vi "Read Waveform Measurement One Channel.vi"(4 "Measurement Type (0: Statistic Average)":u16(ring) items=["Statistic Average", "Current Statistic Value", "Statistic Maximum", "Statistic Minimum", "Statistic Standard Deviation", "Counter"], 6 "Measurement Function (0: Falling Edge)":u16(ring) items=["Waveform Peak-Peak Value", "Waveform Amplitude Value", "Waveform Maximum", "Waveform Minimum", "Waveform Top Value", "Waveform Amplitude Base Value", "Rover Shoot", "Fover Shoot", "RPre Shoot", "FPre Shoot", "Waveform Amplitude Average(Display)", "Waveform Amplitude Average(Cycle)", "Waveform RMS(DC Display)", "Waveform RMS(DC Cycle)", "Waveform RMS(AC Display)", "Waveform RMS(AC Cycle)", "Waveform Adjust Mean", "Period", "Frequency", "Raising Time", "Fall Time", "Positive Pulse", "Negative Pulse", "Positive Duty", "Negative Duty", "Burst Width", "PulSetrain", "XMax", "XMin", "Setup Time", "Hold Time", "ShRatio", "Baud", "Raising Count", "Falling Count", "Positive Count", "Negtive Count", "Triger Count", "Area (Display)", "Area(Cycle)", "Positvie Area(Display)", "Positive Area(Cycle)", "Negtive Area(Display)", "Negtive Area(Cycle)"], 7 "Channel (1: Channel 1)":u16(ring)=1 items=["Channel 1"=1, "Channel 2"=2, "Channel 3"=3, "Channel 4"=4], 8 "error in (no error)":errorcluster, 10 "Timeout (1000 ms)":dbl=1000.0, 11 "VISA resource name":refnum<visa-resource-name>) -> (0 "error out":errorcluster, 2 "Measurement":dbl, 3 "VISA resource name out":refnum<visa-resource-name>)   [LabVIEW 2015, in "ZhiYuan ZDS Series for TCP.lvlib"]
doc: "Returns the waveform the oscilloscope acquired for the specified channel. The waveform is from an acquisition that you initiate prior to calling this VI.\n\nYou use the Initiate VI to start an acquisition on the channels that you enable with the Configure Channel VI. The oscilloscope acquires waveforms for the enabled channels concurrently. You must call this VI separately for each enabled channel to obtain the waveforms.\n\nYou can call the Read Waveform VI instead of using low-level VIs.\n\n<B>Note:</B> Use this VI only with other low-level VIs. The high-level VIs automatically incorporate this functionality. This VI does not check the instrument status."
uses:
  ZhiYuan ZDS Series for TCP.lvlib
panel:
  out "字符串":string
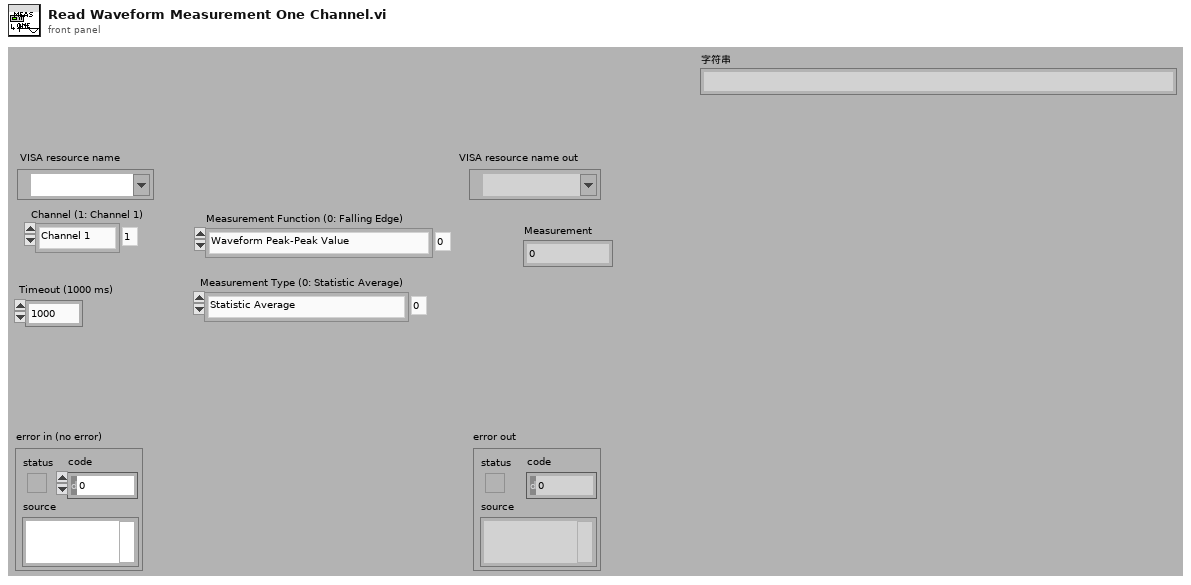
[diagram p1: front panel]
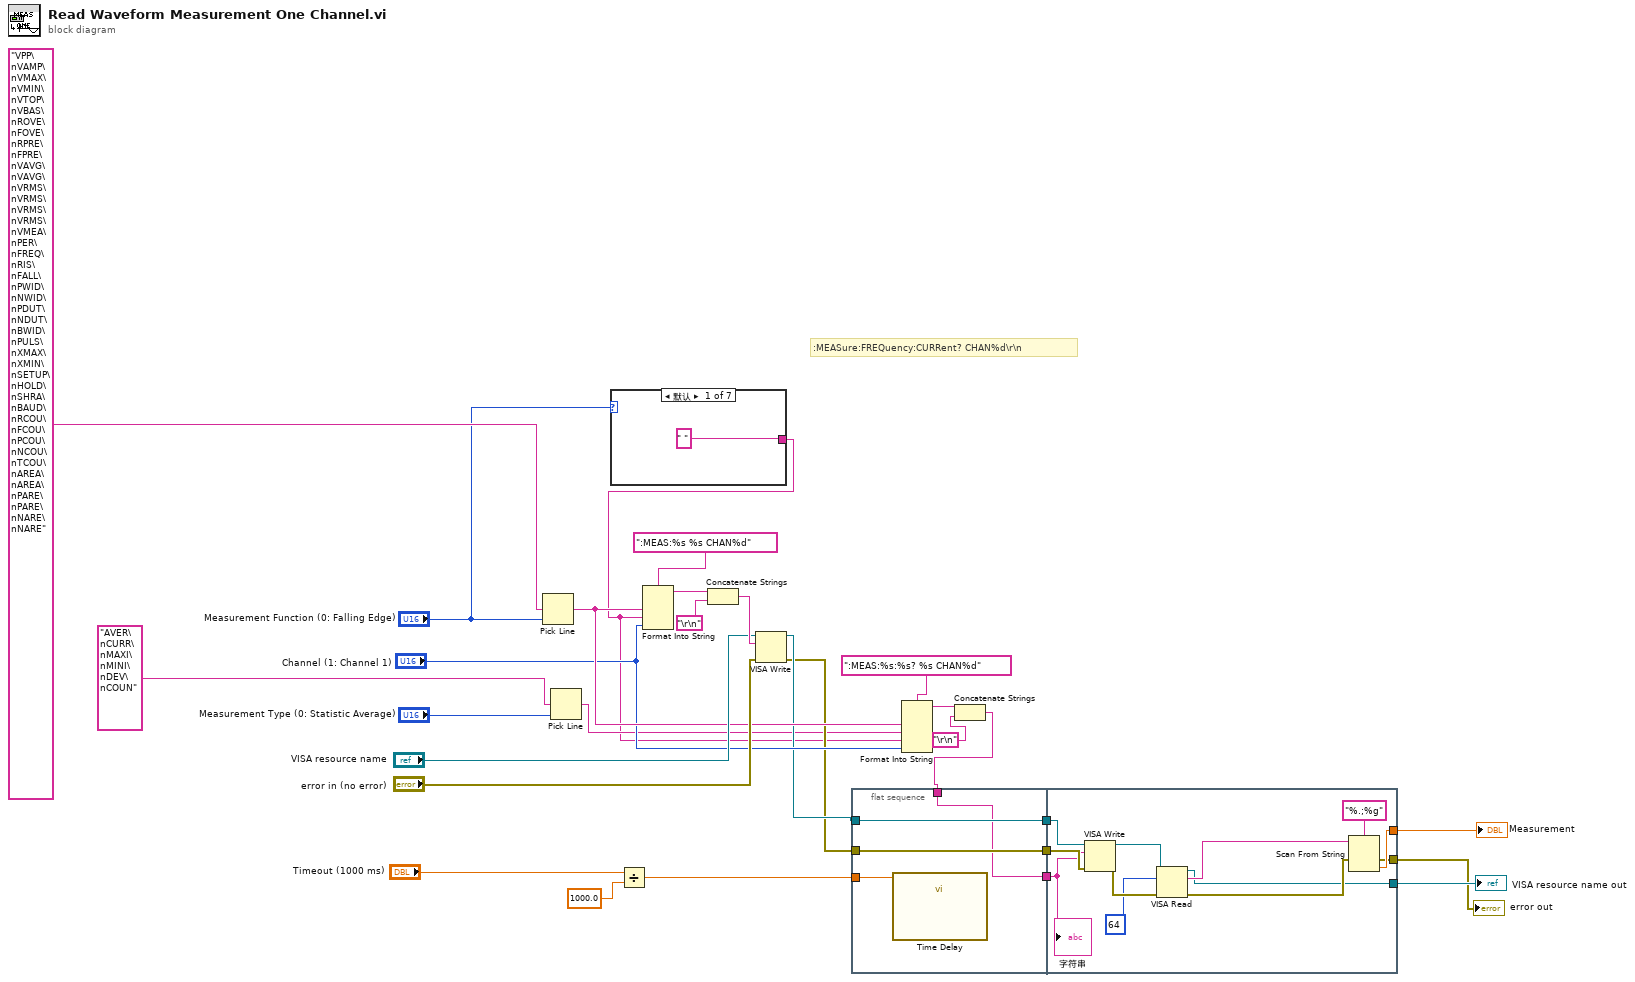
[diagram p0: block diagram]
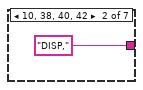
[diagram p2: hidden frame]
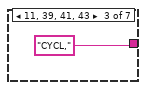
[diagram p3: hidden frame]
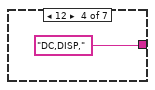
[diagram p4: hidden frame]
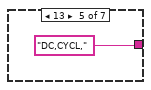
[diagram p5: hidden frame]
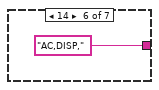
[diagram p6: hidden frame]
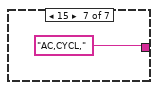
[diagram p7: hidden frame]
diagram:
  # ":MEASure:FREQuency:CURRent? CHAN%d\\r\\n"
  n1 = Pick Line(multi-line string="VPP\nVAMP\nVMAX\nVMIN\nVTOP\nVBAS\nROVE\nFOVE\nRPRE\nFPRE\nVAVG\nVAVG\nVRMS\nVRMS\nVRMS\nVRMS\nVMEA\nPER\nFREQ\nRIS\nFALL\nPWID\nNWID\nPDUT\nNDUT\nBWID\nPULS\nXMAX\nXMIN\nSETUP\nHOLD\nSHRA\nBAUD\nRCOU\nFCOU\nPCOU\nNCOU\nTCOU\nAREA\nAREA\nPARE\nPARE\nNARE\nNARE", line index="Measurement Function (0: Falling Edge)") -> (output string=w18:string)  [unwired: 1 in]
  n2 = Pick Line(multi-line string="AVER\nCURR\nMAXI\nMINI\nDEV\nCOUN", line index="Measurement Type (0: Statistic Average)") -> (output string=w5:string)  [unwired: 1 in]
  n3 = case shown="默认" "Measurement Function (0: Falling Edge)" {
    tunnel: [" " "DISP," "CYCL," "DC,DISP," "DC,CYCL," "AC,DISP," "AC,CYCL,"] -> w4
    frame Default {
    }
    frame 10, 38, 40, 42 {
    }
    frame 11, 39, 41, 43 {
    }
    frame 12 {
    }
    frame 13 {
    }
    frame 14 {
    }
    frame 15 {
    }
  }
  n4 = Divide(x="Timeout (1000 ms)", y=1000.0) -> (x/y=w14:dbl)
  n5 = Format Into String(format string=":MEAS:%s %s CHAN%d" ("write buffer"), w18, w4, "Channel (1: Channel 1)") -> (resulting string=w24:string)  [unwired: 2 in, 1 out]
  n6 = Concatenate Strings(w24, "\r\n") -> (w22:string)
  n7 = VISA Write(VISA resource name="VISA resource name", write buffer=w22, error in (no error)="error in (no error)") -> (VISA resource name out=w12:refnum<visa-resource-name>, error out=w11:errorcluster)  [unwired: 1 out]
  n8 = flat-sequence {
    tunnel: w14 -> [w40]
    tunnel: [w39] -> w13
    tunnel: w12 -> [w39]
    tunnel: w11 -> [w38]
    tunnel: [w38] -> w10
    tunnel: w1 -> [w37]
    tunnel: [w37] -> w9
    tunnel: w13 -> [w47]
    tunnel: w10 -> [w46]
    tunnel: w9 -> [w45]
    tunnel: [w43] -> w8
    tunnel: [w42] -> w7
    tunnel: [w41] -> w6
    frame #0 {
      n9 = call "Time Delay"("Delay Time (s)"=w40) -> ()  [unwired: 10 in, 1 out]
    }
    frame #1 {
      n10 = VISA Write(VISA resource name=w47, write buffer=w45, error in (no error)=w46) -> (VISA resource name out=w49:refnum<visa-resource-name>, error out=w50:errorcluster)  [unwired: 1 out]
      n11 = VISA Read(VISA resource name=w49, byte count=u32 64, error in (no error)=w50) -> (VISA resource name out=w42:refnum<visa-resource-name>, read buffer=w52:string, error out=w44:errorcluster)  [unwired: 1 out]
      n12 = Scan From String(format string="%.;%g", input string=w52, error in=w44) -> (error out=w41:errorcluster, output 1=w43:dbl)  [unwired: 2 in, 2 out]
      "字符串" <- w45
    }
  }
  n13 = Format Into String(format string=":MEAS:%s:%s? %s CHAN%d" ("write buffer"), w18, w5, w4, "Channel (1: Channel 1)") -> (resulting string=w3:string)  [unwired: 2 in, 1 out]
  n14 = Concatenate Strings(w3, "\r\n") -> (w1:string)
  "Measurement" <- w8
  "VISA resource name out" <- w7
  "error out" <- w6
